vi "HardwareLoop.vi"(8 "Error In":errorcluster, 11 "Action Queues":T1) -> (0 "Error Out":errorcluster)   [LabVIEW 2012]
uses:
  ActionQueues.ctl
  UIActionQueueElement.ctl
  UIAction.ctl
  HardwareActionQueueElement.ctl
  HardwareAction.ctl
  driver/Public/Controls/Pattern.ctl
  driver/Public/Controls/Input.ctl
  driver/Virtual-PGA.lvlib
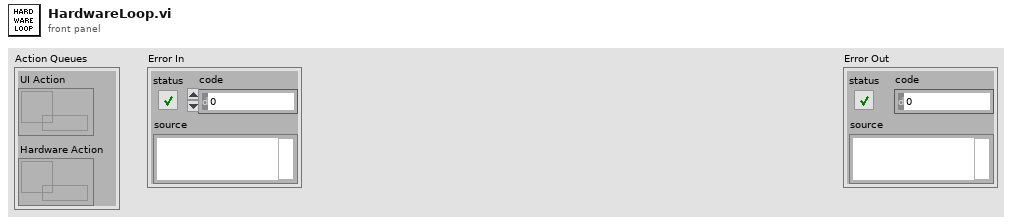
[diagram p1: front panel]
types:
  T1 = typedef "ActionQueues.ctl" = cluster{"UI Action":refnum<queue>, "Hardware Action":refnum<queue>}
  T2 = typedef "UIActionQueueElement.ctl" = cluster{"Action":T3, "Data":variant}
  T3 = typedef "UIAction.ctl" = enum16{"Initialize", "Connected", "Select Pattern", "Update Patterns", "Error", "Shutdown"}
  T4 = typedef "HardwareActionQueueElement.ctl" = cluster{"State":T5, "Data":variant}
  T5 = typedef "HardwareAction.ctl" = enum16{"Initialize", "Start", "Read", "Write", "Stop", "Shutdown"}
  T6 = typedef "Virtual-PGA.lvlib/Pattern.ctl" = cluster{"Name":string, "Description":string, "Inputs":T7[]}
  T7 = typedef "Virtual-PGA.lvlib/Input.ctl" = cluster{"ID":string, "Label":string, "Pads":u32[]}
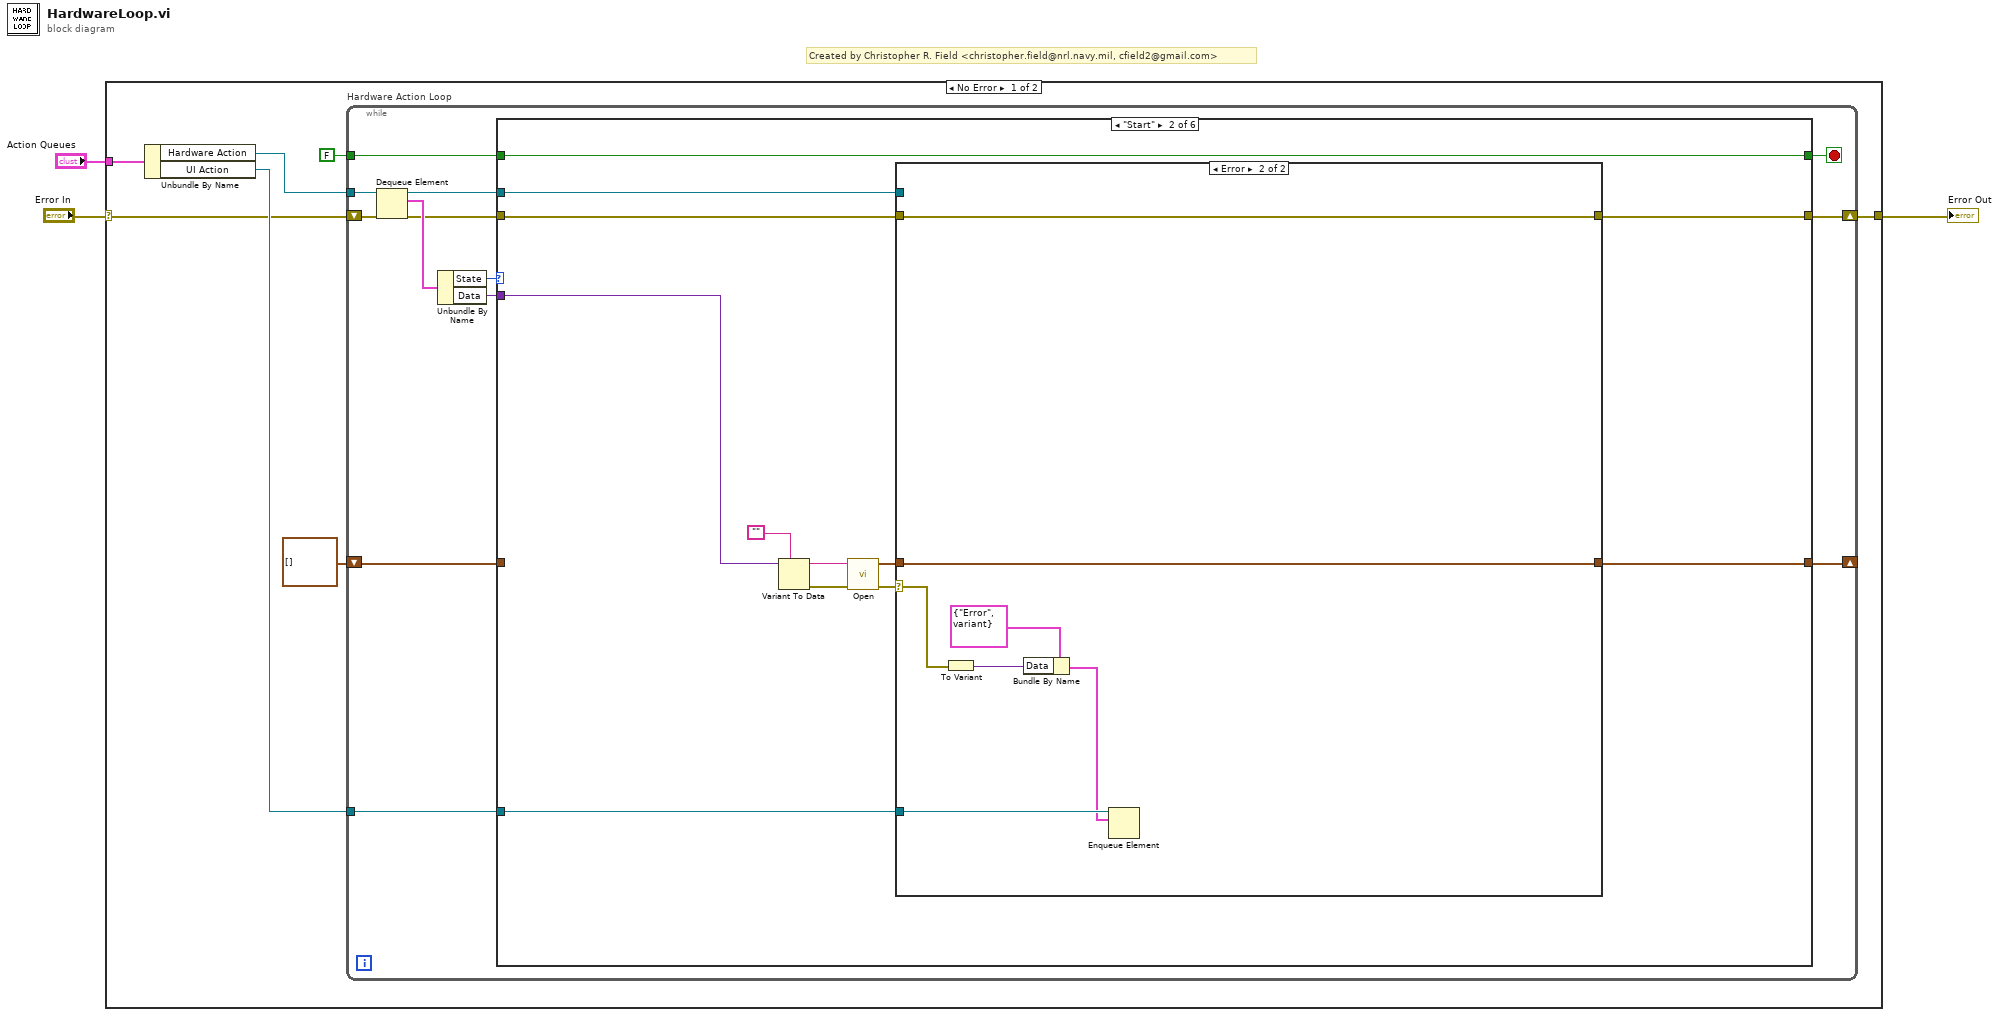
[diagram p0: block diagram]
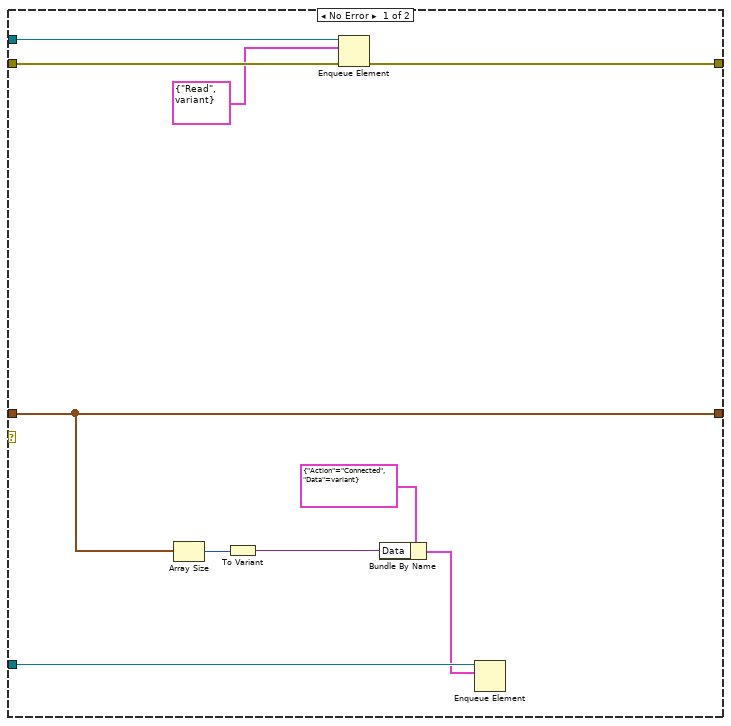
[diagram p3: hidden frame]
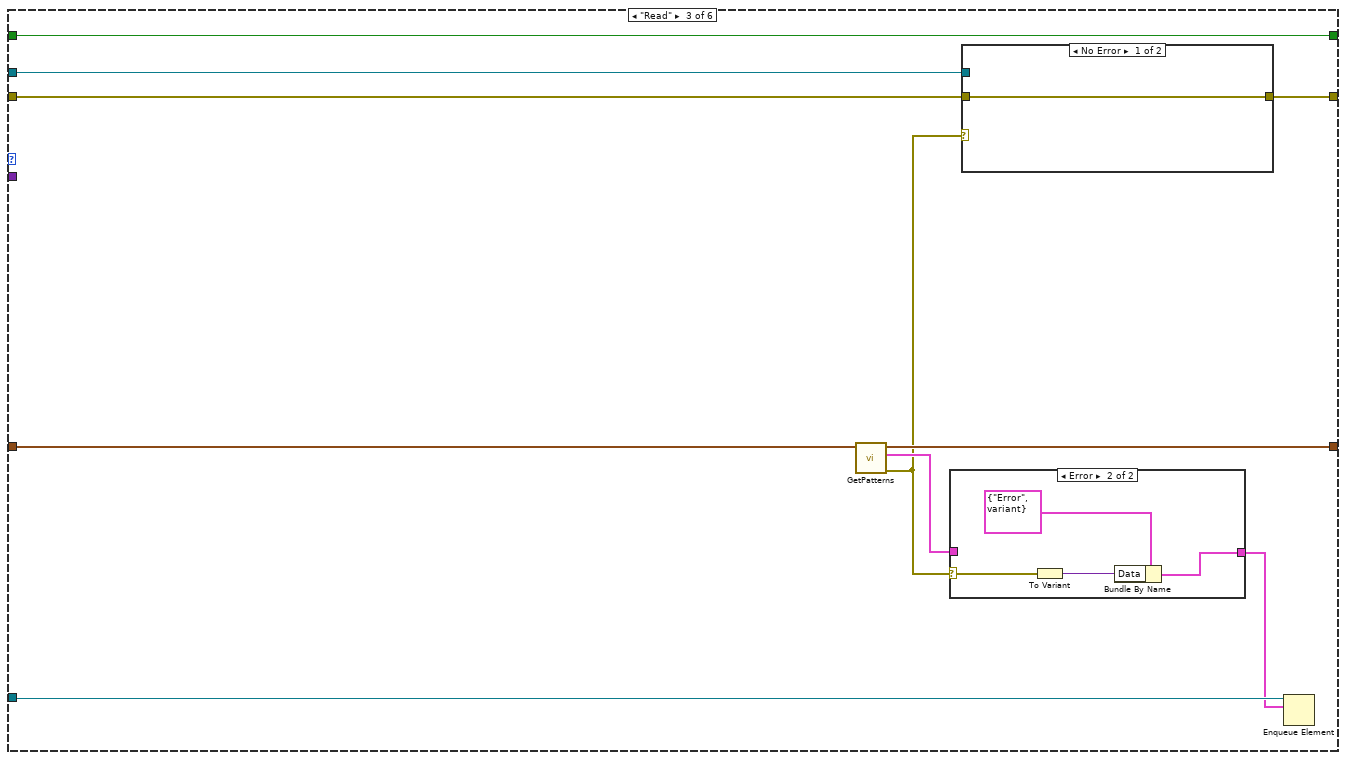
[diagram p4: hidden frame]
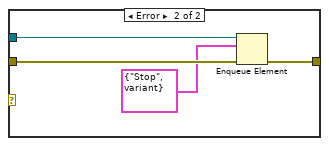
[diagram p5: hidden frame]
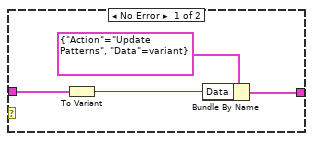
[diagram p6: hidden frame]
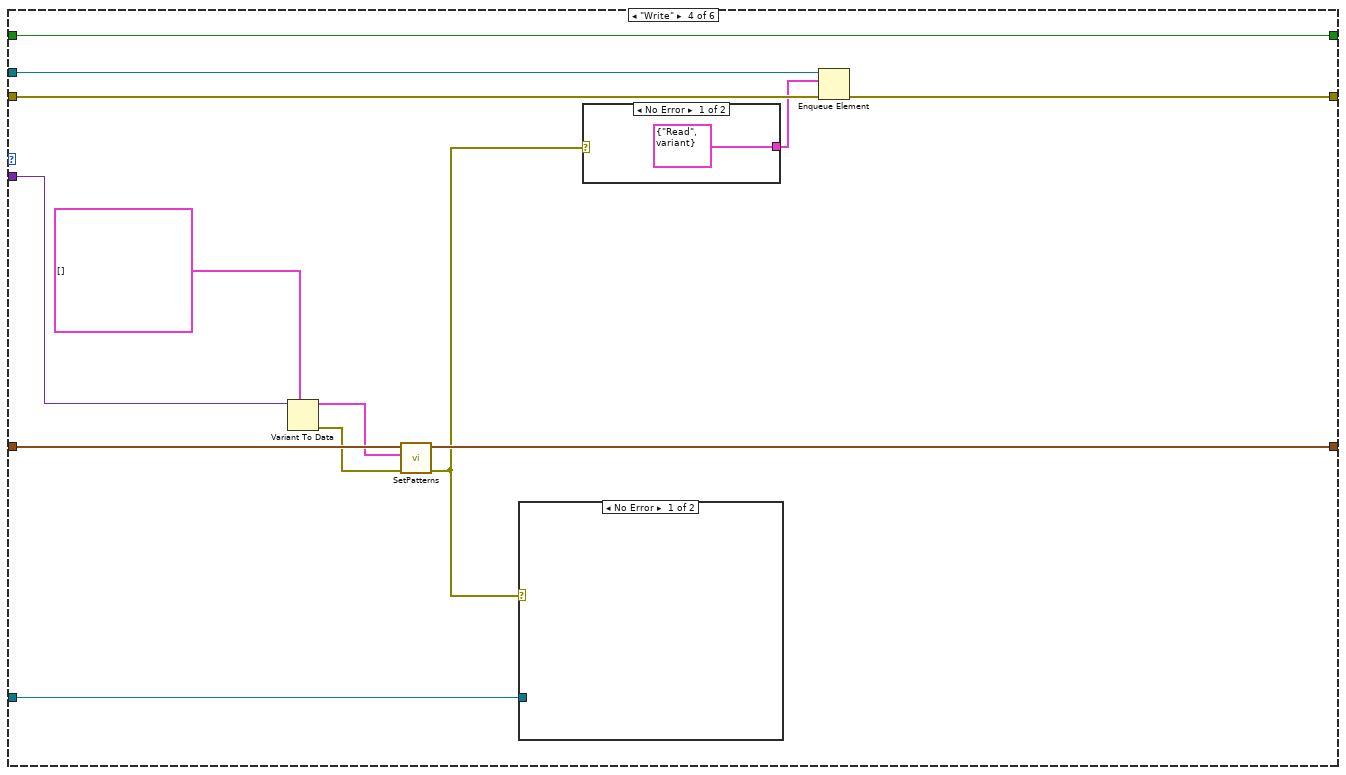
[diagram p7: hidden frame]
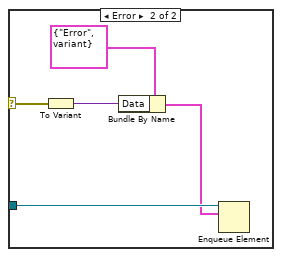
[diagram p8: hidden frame]
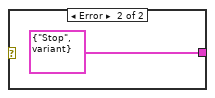
[diagram p9: hidden frame]
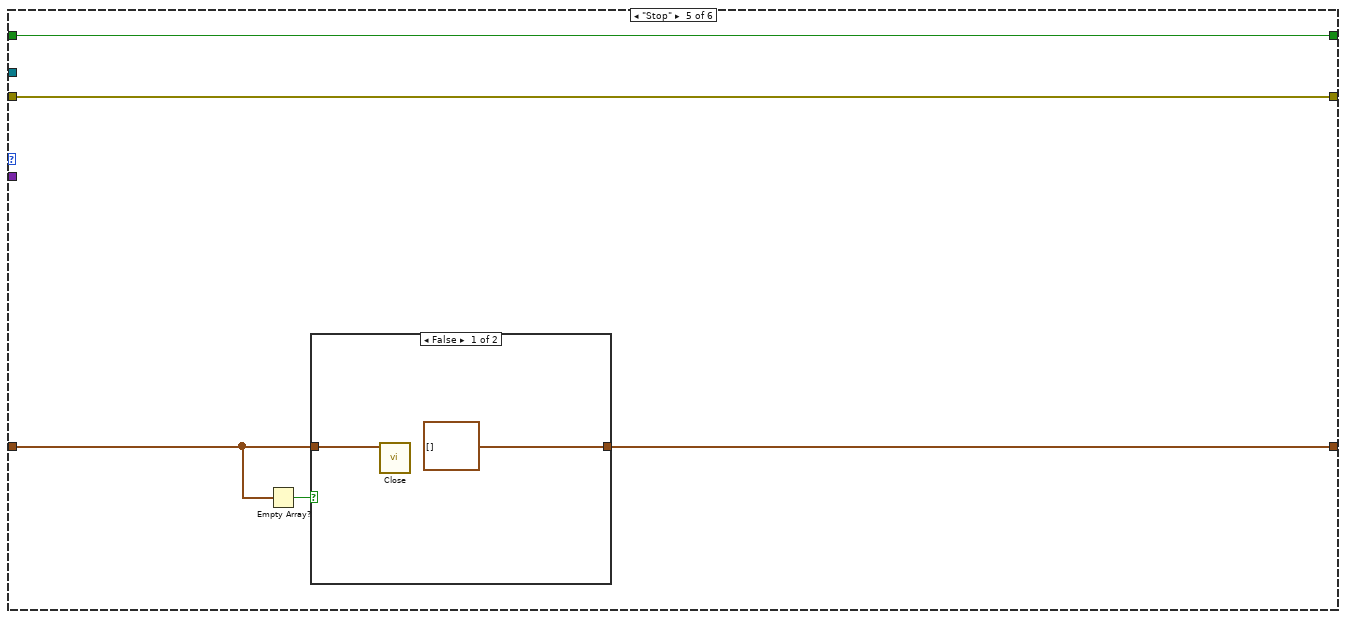
[diagram p10: hidden frame]
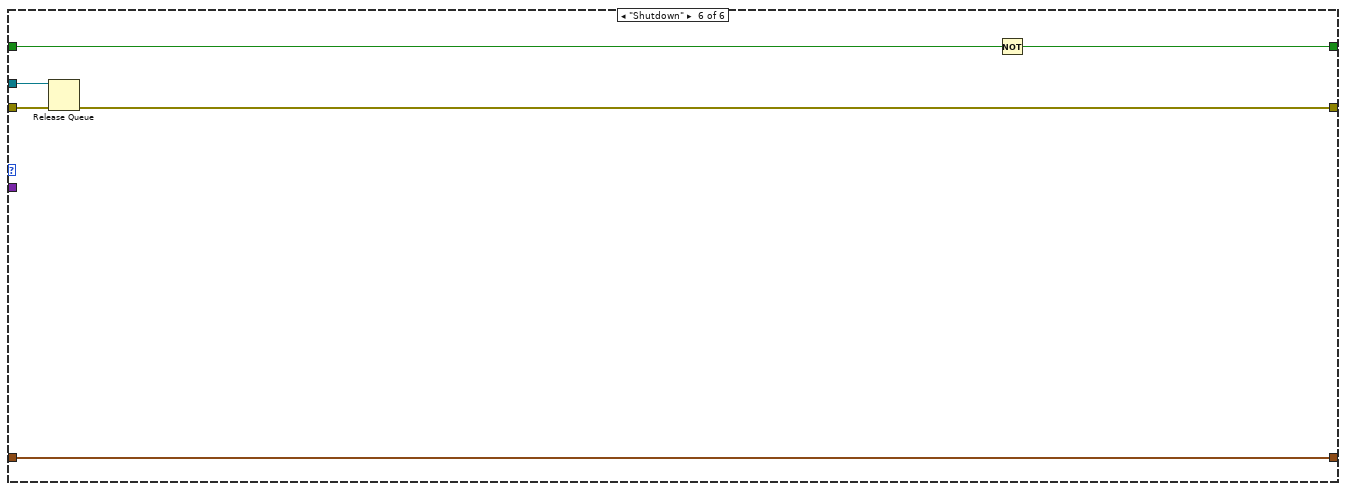
[diagram p12: hidden frame]
diagram:
  # "Created by Christopher R. Field <christopher.field@nrl.navy.mil, cfield2@gmail.com>"
  n1 = case shown="No Error" "Error In" {
    selector: "Error In" -> [w4 w113]
    tunnel: "Action Queues" -> [w10 _]
    tunnel: [w7 w113] -> w2
    frame No Error {
      n2 = Unbundle By Name(w10) -> ("Hardware Action"=w9:refnum<queue>, "UI Action"=w8:refnum<queue>)
      n3 = while "Hardware Action Loop" {
        tunnel: w9 -> [w23]
        tunnel: FALSE -> [w15]
        tunnel: w8 -> [w11]
        shift-right: [w16] -> w7
        shift-left: w4 -> [w17]
        shift-right: [w13] -> _
        shift-left: cluster{"Session":u32, "Card number":u32}[] [] ("Switch Out") -> [w12]
        stop <- w14 stop-if-true
        n4 = Dequeue Element(queue=w23, error in (no error)=w17) -> (queue out=w22:refnum<queue>, element=w21:T4, error out=w20:errorcluster)  [unwired: 1 in, 1 out]
        n5 = Unbundle By Name(w21) -> ("State"=w19:T5, "Data"=w18:variant)
        n6 = case shown="\"Start\"" w19 {
          tunnel: w22 -> [_ w32 w61 w85 _ w110]
          tunnel: w20 -> [w26 w34 w62 w86 w102 w109]
          tunnel: w18 -> [_ w37 _ w88 _ _]
          tunnel: [w26 w31 w60 w84 w102 w108] -> w16
          tunnel: w15 -> [w25 w38 w65 w91 w103 w112]
          tunnel: [w25 w38 w65 w91 w103 w111] -> w14
          tunnel: [w24 w30 w57 w89 w101 w107] -> w13
          tunnel: w12 -> [w24 _ w59 w90 w99 w107]
          tunnel: w11 -> [_ w29 w64 w81 _ _]
          frame "Initialize", Default {
          }
          frame "Start" {
            n7 = Variant To Data(type="", Variant=w37) -> (data=w27:string, error out=w36:errorcluster)  [unwired: 1 in]
            n8 = call "Open.vi"("Error In"=w36, "IP Address"=w27) -> ("Error Out"=w35:errorcluster, "Cards Out"=w33:cluster{"Session":u32, "Card number":u32}[])  [unwired: 8 in]
            n9 = case shown="Error" w35 {
              selector: w35 -> [_ w52]
              tunnel: w34 -> [w48 w54]
              tunnel: w33 -> [w43 w55]
              tunnel: w32 -> [w47 _]
              tunnel: [w46 w54] -> w31
              tunnel: [w43 w55] -> w30
              tunnel: w29 -> [w44 w50]
              frame No Error {
                n10 = Array Size(array=w43) -> (size(s)=w42:i32)
                n11 = To Variant(anything=w42) -> (Variant=w40:variant)
                n12 = Enqueue Element(queue=w47, element=T4 {"State"=enum."Read", "Data"=variant} ("Acquisition Queue Element"), error in (no error)=w48) -> (error out=w46:errorcluster)  [unwired: 1 in, 2 out]
                n13 = Bundle By Name(cluster=T2 {"Action"=enum."Connected", "Data"=variant} ("User Interface Queue Element"), "Data"=w40) -> (w39:T2)
                n14 = Enqueue Element(queue=w44, element=w39) -> ()  [unwired: 2 in, 3 out]
              }
              frame Error {
                n15 = To Variant(anything=w52) -> (Variant=w51:variant)
                n16 = Bundle By Name(cluster=T2 {"Action"=enum."Error", "Data"=variant} ("User Interface Queue Element"), "Data"=w51) -> (w49:T2)
                n17 = Enqueue Element(queue=w50, element=w49) -> ()  [unwired: 2 in, 3 out]
              }
            }
          }
          frame "Read" {
            n18 = call "GetPatterns.vi"("Cards In"=w59) -> ("Error Out"=w56:errorcluster, "Patterns"=w58:T6[], "Cards Out"=w57:cluster{"Session":u32, "Card number":u32}[])  [unwired: 8 in]
            n19 = case shown="Error" w56 {
              selector: w56 -> [_ w77]
              tunnel: [w72 w75] -> w63
              tunnel: w58 -> [w71 _]
              frame No Error {
                n20 = To Variant(anything=w71) -> (Variant=w73:variant)
                n21 = Bundle By Name(cluster=T2 {"Action"=enum."Update Patterns", "Data"=variant} ("User Interface Queue Element"), "Data"=w73) -> (w72:T2)
              }
              frame Error {
                n22 = To Variant(anything=w77) -> (Variant=w76:variant)
                n23 = Bundle By Name(cluster=T2 {"Action"=enum."Error", "Data"=variant} ("User Interface Queue Element"), "Data"=w76) -> (w75:T2)
              }
            }
            n24 = case shown="No Error" w56 {
              tunnel: w62 -> [w66 w69]
              tunnel: w61 -> [_ w70]
              tunnel: [w66 w67] -> w60
              frame No Error {
              }
              frame Error {
                n25 = Enqueue Element(queue=w70, element=T4 {"State"=enum."Stop", "Data"=variant}, error in (no error)=w69) -> (error out=w67:errorcluster)  [unwired: 1 in, 2 out]
              }
            }
            n26 = Enqueue Element(queue=w64, element=w63) -> ()  [unwired: 2 in, 3 out]
          }
          frame "Write" {
            n27 = Variant To Data(type=T6[] [], Variant=w88) -> (data=w79:T6[], error out=w87:errorcluster)  [unwired: 1 in]
            n28 = call "SetPatterns.vi"("Error In"=w87, "Patterns"=w79, "Cards In"=w90) -> ("Error Out"=w82:errorcluster, "Cards Out"=w89:cluster{"Session":u32, "Card number":u32}[])  [unwired: 7 in]
            n29 = case shown="No Error" w82 {
              selector: w82 -> [_ w94]
              tunnel: w81 -> [_ w96]
              frame No Error {
              }
              frame Error {
                n30 = To Variant(anything=w94) -> (Variant=w93:variant)
                n31 = Bundle By Name(cluster=T2 {"Action"=enum."Error", "Data"=variant} ("User Interface Queue Element"), "Data"=w93) -> (w92:T2)
                n32 = Enqueue Element(queue=w96, element=w92) -> ()  [unwired: 2 in, 3 out]
              }
            }
            n33 = case shown="No Error" w82 {
              tunnel: [T4 {"State"=enum."Read", "Data"=variant} ("element") T4 {"State"=enum."Stop", "Data"=variant} ("element")] -> w83
              frame No Error {
              }
              frame Error {
              }
            }
            n34 = Enqueue Element(queue=w85, element=w83, error in (no error)=w86) -> (error out=w84:errorcluster)  [unwired: 1 in, 2 out]
          }
          frame "Stop" {
            n35 = Empty Array?(array=w99) -> (empty?=w100:bool)
            n36 = case shown="False" w100 {
              tunnel: w99 -> [w105 w106]
              tunnel: [cluster{"Session":u32, "Card number":u32}[] [] ("Switch Out") w106] -> w101
              frame False {
                n37 = call "Close.vi"("Cards In"=w105) -> ()  [unwired: 10 in, 1 out]
              }
              frame True {
              }
            }
          }
          frame "Shutdown" {
            n38 = Release Queue(queue=w110, error in (no error)=w109) -> (error out=w108:errorcluster)  [unwired: 1 in, 2 out]
            n39 = Not(x=w112) -> (.not. x?=w111:bool)
          }
        }
      }
    }
    frame Error {
    }
  }
  "Error Out" <- w2
